vi "canDataSort.vi"() -> ()   [LabVIEW 2023] (continued)
8        68\t00\t97\tCC\t00\t19\t39\tFB\r\n      4502  1FFFFFFF   00000004    8        00\t00\tFF\tFF\tFF\tFF\tFF\tFF\r\n      4493  18F106A7   00000004    8        00\tF7\tFF\tFF\tFF\tFF\tFF\tCA\r\n      4492  1FFFFFFF   00000004    8        00\t20\tFF\tFF\tFF\tFF\tFF\tFF\r\n      4483  0CF102A7   00000004    8        30\t75\tE0\t2E\t80\tFF\tFF\tFD\r\n      4482  0CF101A7   00000004    8        68\t00\t97\tCC\t00\t19\t39\tFA\r\n      4482  1FFFFFFF   00000004    8        00\t00\tFF\tFF\tFF\tFF\tFF\tFF\r\n      4472  1FFFFFFF   00000004    8        00\t00\tFF\tFF\tFF\tFF\tFF\tFF\r\n      4463  0CF102A7   00000004    8        30\t75\tE0\t2E\t80\tFF\tFF\tFD\r\n      4463  0CF101A7   00000004    8        68\t00\t97\tCC\t00\t19\t39\tF9\r\n      4462  1FFFFFFF   00000004    8        00\t00\tFF\tFF\tFF\tFF\tFF\tFF\r\n      4503  0CF102A7   00000004    8        30\t75\tE0\t2E\t80\tFF\tFF\tFD\r\n      4503  0CF101A7   00000004    8        68\t00\t97\tCC\t00\t19\t39\tFB\r\n      4502  1FFFFFFF   00000004    8        00\t00\tFF\tFF\tFF\tFF\tFF\tFF\r\n      4493  18F106A7   00000004    8        00\tF7\tFF\tFF\tFF\tFF\tFF\tCA\r\n      4492  1FFFFFFF   00000004    8        00\t20\tFF\tFF\tFF\tFF\tFF\tFF\r\n      4483  0CF102A7   00000004    8        30\t75\tE0\t2E\t80\tFF\tFF\tFD\r\n      4482  0CF101A7   00000004    8        68\t00\t97\tCC\t00\t19\t39\tFA\r\n      4482  1FFFFFFF   00000004    8        00\t00\tFF\tFF\tFF\tFF\tFF\tFF\r\n      4472  1FFFFFFF   00000004    8        00\t00\tFF\tFF\tFF\tFF\tFF\tFF\r\n      4463  0CF102A7   00000004    8        30\t75\tE0\t2E\t80\tFF\tFF\tFD\r\n      4463  0CF101A7   00000004    8        68\t00\t97\tCC\t00\t19\t39\tF9\r\n      4512  1FFFFFFF   00000004    8        00\t00\tFF\tFF\tFF\tFF\tFF\tFF\r\n      4503  0CF102A7   00000004    8        30\t75\tE0\t2E\t80\tFF\tFF\tFD\r\n      4503  0CF101A7   00000004    8        68\t00\t97\tCC\t00\t19\t39\tFB\r\n      4502  1FFFFFFF   00000004    8        00\t00\tFF\tFF\tFF\tFF\tFF\tFF\r\n      4493  18F106A7   00000004    8        00\tF7\tFF\tFF\tFF\tFF\tFF\tCA\r\n      4492  1FFFFFFF   00000004    8        00\t20\tFF\tFF\tFF\tFF\tFF\tFF\r\n      4483  0CF102A7   00000004    8        30\t75\tE0\t2E\t80\tFF\tFF\tFD\r\n      4482  0CF101A7   00000004    8        68\t00\t97\tCC\t00\t19\t39\tFA\r\n      4482  1FFFFFFF   00000004    8        00\t00\tFF\tFF\tFF\tFF\tFF\tFF\r\n      4472  1FFFFFFF   00000004    8        00\t00\tFF\tFF\tFF\tFF\tFF\tFF\r\n      4463  0CF102A7   00000004    8        30\t75\tE0\t2E\t80\tFF\tFF\tFD\r\n      4522  1FFFFFFF   00000004    8        00\t00\tFF\tFF\tFF\tFF\tFF\tFF\r\n      4512  1FFFFFFF   00000004    8        00\t00\tFF\tFF\tFF\tFF\tFF\tFF\r\n      4503  0CF102A7   00000004    8        30\t75\tE0\t2E\t80\tFF\tFF\tFD\r\n      4503  0CF101A7   00000004    8        68\t00\t97\tCC\t00\t19\t39\tFB\r\n      4502  1FFFFFFF   00000004    8        00\t00\tFF\tFF\tFF\tFF\tFF\tFF\r\n      4493  18F106A7   00000004    8        00\tF7\tFF\tFF\tFF\tFF\tFF\tCA\r\n      4492  1FFFFFFF   00000004    8        00\t20\tFF\tFF\tFF\tFF\tFF\tFF\r\n      4483  0CF102A7   00000004    8        30\t75\tE0\t2E\t80\tFF\tFF\tFD\r\n      4482  0CF101A7   00000004    8        68\t00\t97\tCC\t00\t19\t39\tFA\r\n      4482  1FFFFFFF   00000004    8        00\t00\tFF\tFF\tFF\tFF\tFF\tFF\r\n      4472  1FFFFFFF   00000004    8        00\t00\tFF\tFF\tFF\tFF\tFF\tFF\r\n      4523  0CF101A7   00000004    8        68\t00\t97\tCC\t00\t19\t39\tFC\r\n      4522  1FFFFFFF   00000004    8        00\t00\tFF\tFF\tFF\tFF\tFF\tFF\r\n      4512  1FFFFFFF   00000004    8        00\t00\tFF\tFF\tFF\tFF\tFF\tFF\r\n      4503  0CF102A7   00000004    8        30\t75\tE0\t2E\t80\tFF\tFF\tFD\r\n      4503  0CF101A7   00000004    8        68\t00\t97\tCC\t00\t19\t39\tFB\r\n      4502  1FFFFFFF   00000004    8        00\t00\tFF\tFF\tFF\tFF\tFF\tFF\r\n      4493  18F106A7   00000004    8        00\tF7\tFF\tFF\tFF\tFF\tFF\tCA\r\n      4492  1FFFFFFF   00000004    8        00\t20\tFF\tFF\tFF\tFF\tFF\tFF\r\n      4483  0CF102A7   00000004    8        30\t75\tE0\t2E\t80\tFF\tFF\tFD\r\n      4482  0CF101A7   00000004    8        68\t00\t97\tCC\t00\t19\t39\tFA\r\n      4482  1FFFFFFF   00000004    8        00\t00\tFF\tFF\tFF\tFF\tFF\tFF\r\n      4523  0CF102A7   00000004    8        30\t75\tE0\t2E\t80\tFF\tFF\tFD\r\n      4523  0CF101A7   00000004    8        68\t00\t97\tCC\t00\t19\t39\tFC\r\n      4522  1FFFFFFF   00000004    8        00\t00\tFF\tFF\tFF\tFF\tFF\tFF\r\n      4512  1FFFFFFF   00000004    8        00\t00\tFF\tFF\tFF\tFF\tFF\tFF\r\n      4503  0CF102A7   00000004    8        30\t75\tE0\t2E\t80\tFF\tFF\tFD\r\n      4503  0CF101A7   00000004    8        68\t00\t97\tCC\t00\t19\t39\tFB\r\n      4502  1FFFFFFF   00000004    8        00\t00\tFF\tFF\tFF\tFF\tFF\tFF\r\n      4493  18F106A7   00000004    8        00\tF7\tFF\tFF\tFF\tFF\tFF\tCA\r\n      4492  1FFFFFFF   00000004    8        00\t20\tFF\tFF\tFF\tFF\tFF\tFF\r\n      4483  0CF102A7   00000004    8        30\t75\tE0\t2E\t80\tFF\tFF\tFD\r\n      4482  0CF101A7   00000004    8        68\t00\t97\tCC\t00\t19\t39\tFA\r\n      4532  1FFFFFFF   00000004    8        00\t20\tFF\tFF\tFF\tFF\tFF\tFF\r\n      4523  0CF102A7   00000004    8        30\t75\tE0\t2E\t80\tFF\tFF\tFD\r\n      4523  0CF101A7   00000004    8        68\t00\t97\tCC\t00\t19\t39\tFC\r\n      4522  1FFFFFFF   00000004    8        00\t00\tFF\tFF\tFF\tFF\tFF\tFF\r\n      4512  1FFFFFFF   00000004    8        00\t00\tFF\tFF\tFF\tFF\tFF\tFF\r\n      4503  0CF102A7   00000004    8        30\t75\tE0\t2E\t80\tFF\tFF\tFD\r\n      4503  0CF101A7   00000004    8        68\t00\t97\tCC\t00\t19\t39\tFB\r\n      4502  1FFFFFFF   00000004    8        00\t00\tFF\tFF\tFF\tFF\tFF\tFF\r\n      4493  18F106A7   00000004    8        00\tF7\tFF\tFF\tFF\tFF\tFF\tCA\r\n      4492  1FFFFFFF   00000004    8        00\t20\tFF\tFF\tFF\tFF\tFF\tFF\r\n      4483  0CF102A7   00000004    8        30\t75\tE0\t2E\t80\tFF\tFF\tFD\r\n      4541  18F11FF0   00000004    8        FF\t3F\t90\t68\t88\t1B\t10\t5C\r\n      4532  1FFFFFFF   00000004    8        00\t20\tFF\tFF\tFF\tFF\tFF\tFF\r\n      4523  0CF102A7   00000004    8        30\t75\tE0\t2E\t80\tFF\tFF\tFD\r\n      4523  0CF101A7   00000004    8        68\t00\t97\tCC\t00\t19\t39\tFC\r\n      4522  1FFFFFFF   00000004    8        00\t00\tFF\tFF\tFF\tFF\tFF\tFF\r\n      4512  1FFFFFFF   00000004    8        00\t00\tFF\tFF\tFF\tFF\tFF\tFF\r\n      4503  0CF102A7   00000004    8        30\t75\tE0\t2E\t80\tFF\tFF\tFD\r\n      4503  0CF101A7   00000004    8        68\t00\t97\tCC\t00\t19\t39\tFB\r\n      4502  1FFFFFFF   00000004    8        00\t00\tFF\tFF\tFF\tFF\tFF\tFF\r\n      4493  18F106A7   00000004    8        00\tF7\tFF\tFF\tFF\tFF\tFF\tCA\r\n      4492  1FFFFFFF   00000004    8        00\t20\tFF\tFF\tFF\tFF\tFF\tFF\r\n      4542  18F120F0   00000004    8        2B\t75\t60\tB1\tB0\t01\tFF\tFF\r\n      4541  18F11FF0   00000004    8        FF\t3F\t90\t68\t88\t1B\t10\t5C\r\n      4532  1FFFFFFF   00000004    8        00\t20\tFF\tFF\tFF\tFF\tFF\tFF\r\n      4523  0CF102A7   00000004    8        30\t75\tE0\t2E\t80\tFF\tFF\tFD\r\n      4523  0CF101A7   00000004    8        68\t00\t97\tCC\t00\t19\t39\tFC\r\n      4522  1FFFFFFF   00000004    8        00\t00\tFF\tFF\tFF\tFF\tFF\tFF\r\n      4512  1FFFFFFF   00000004    8        00\t00\tFF\tFF\tFF\tFF\tFF\tFF\r\n      4503  0CF102A7   00000004    8        30\t75\tE0\t2E\t80\tFF\tFF\tFD\r\n      4503  0CF101A7   00000004    8        68\t00\t97\tCC\t00\t19\t39\tFB\r\n      4502  1FFFFFFF   00000004    8        00\t00\tFF\tFF\tFF\tFF\tFF\tFF\r\n      4493  18F106A7   00000004    8        00\tF7\tFF\tFF\tFF\tFF\tFF\tCA\r\n      4542  0CF101A7   00000004    8        68\t00\t97\tCC\t00\t19\t39\tFD\r\n      4542  18F120F0   00000004    8        2B\t75\t60\tB1\tB0\t01\tFF\tFF\r\n      4541  18F11FF0   00000004    8        FF\t3F\t90\t68\t88\t1B\t10\t5C\r\n      4532  1FFFFFFF   00000004    8        00\t20\tFF\tFF\tFF\tFF\tFF\tFF\r\n      4523  0CF102A7   00000004    8        30\t75\tE0\t2E\t80\tFF\tFF\tFD\r\n      4523  0CF101A7   00000004    8        68\t00\t97\tCC\t00\t19\t39\tFC\r\n      4522  1FFFFFFF   00000004    8        00\t00\tFF\tFF\tFF\tFF\tFF\tFF\r\n      4512  1FFFFFFF   00000004    8        00\t00\tFF\tFF\tFF\tFF\tFF\tFF\r\n      4503  0CF102A7   00000004    8        30\t75\tE0\t2E\t80\tFF\tFF\tFD\r\n      4503  0CF101A7   00000004    8        68\t00\t97\tCC\t00\t19\t39\tFB\r\n      4502  1FFFFFFF   00000004    8        00\t00\tFF\tFF\tFF\tFF\tFF\tFF\r\n      4543  0C3C4D4A   00000004    8        BE\tFF\tFF\t7F\t18\tFF\tFF\t65\r\n      4542  0CF101A7   00000004    8        68\t00\t97\tCC\t00\t19\t39\tFD\r\n      4542  18F120F0   00000004    8        2B\t75\t60\tB1\tB0\t01\tFF\tFF\r\n      4541  18F11FF0   00000004    8        FF\t3F\t90\t68\t88\t1B\t10\t5C\r\n      4532  1FFFFFFF   00000004    8        00\t20\tFF\tFF\tFF\tFF\tFF\tFF\r\n      4523  0CF102A7   00000004    8        30\t75\tE0\t2E\t80\tFF\tFF\tFD\r\n      4523  0CF101A7   00000004    8        68\t00\t97\tCC\t00\t19\t39\tFC\r\n      4522  1FFFFFFF   00000004    8        00\t00\tFF\tFF\tFF\tFF\tFF\tFF\r\n      4512  1FFFFFFF   00000004    8        00\t00\tFF\tFF\tFF\tFF\tFF\tFF\r\n      4503  0CF102A7   00000004    8        30\t75\tE0\t2E\t80\tFF\tFF\tFD\r\n      4503  0CF101A7   00000004    8        68\t00\t97\tCC\t00\t19\t39\tFB\r\n      4544  0CF102A7   00000004    8        30\t75\tE0\t2E\t80\tFF\tFF\tFD\r\n      4543  0C3C4D4A   00000004    8        BE\tFF\tFF\t7F\t18\tFF\tFF\t65\r\n      4542  0CF101A7   00000004    8        68\t00\t97\tCC\t00\t19\t39\tFD\r\n      4542  18F120F0   00000004    8        2B\t75\t60\tB1\tB0\t01\tFF\tFF\r\n      4541  18F11FF0   00000004    8        FF\t3F\t90\t68\t88\t1B\t10\t5C\r\n      4532  1FFFFFFF   00000004    8        00\t20\tFF\tFF\tFF\tFF\tFF\tFF\r\n      4523  0CF102A7   00000004    8        30\t75\tE0\t2E\t80\tFF\tFF\tFD\r\n      4523  0CF101A7   00000004    8        68\t00\t97\tCC\t00\t19\t39\tFC\r\n      4522  1FFFFFFF   00000004    8        00\t00\tFF\tFF\tFF\tFF\tFF\tFF\r\n      4512  1FFFFFFF   00000004    8        00\t00\tFF\tFF\tFF\tFF\tFF\tFF\r\n      4503  0CF102A7   00000004    8        30\t75\tE0\t2E\t80\tFF\tFF\tFD\r\n      4544  0CF103A7   00000004    8        17\t1F\t08\t60\tB1\t1F\t08\t65\r\n      4544  0CF102A7   00000004    8        30\t75\tE0\t2E\t80\tFF\tFF\tFD\r\n      4543  0C3C4D4A   00000004    8        BE\tFF\tFF\t7F\t18\tFF\tFF\t65\r\n      4542  0CF101A7   00000004    8        68\t00\t97\tCC\t00\t19\t39\tFD\r\n      4542  18F120F0   00000004    8        2B\t75\t60\tB1\tB0\t01\tFF\tFF\r\n      4541  18F11FF0   00000004    8        FF\t3F\t90\t68\t88\t1B\t10\t5C\r\n      4532  1FFFFFFF   00000004    8        00\t20\tFF\tFF\tFF\tFF\tFF\tFF\r\n      4523  0CF102A7   00000004    8        30\t75\tE0\t2E\t80\tFF\tFF\tFD\r\n      4523  0CF101A7   00000004    8        68\t00\t97\tCC\t00\t19\t39\tFC\r\n      4522  1FFFFFFF   00000004    8        00\t00\tFF\tFF\tFF\tFF\tFF\tFF\r\n      4512  1FFFFFFF   00000004    8        00\t00\tFF\tFF\tFF\tFF\tFF\tFF\r\n      4545  0CF104A7   00000004    8        F0\t60\t22\tFC\tFF\tFF\tFF\t65\r\n      4544  0CF103A7   00000004    8        17\t1F\t08\t60\tB1\t1F\t08\t65\r\n      4544  0CF102A7   00000004    8        30\t75\tE0\t2E\t80\tFF\tFF\tFD\r\n      4543  0C3C4D4A   00000004    8        BE\tFF\tFF\t7F\t18\tFF\tFF\t65\r\n      4542  0CF101A7   00000004    8        68\t00\t97\tCC\t00\t19\t39\tFD\r\n      4542  18F120F0   00000004    8        2B\t75\t60\tB1\tB0\t01\tFF\tFF\r\n      4541  18F11FF0   00000004    8        FF\t3F\t90\t68\t88\t1B\t10\t5C\r\n      4532  1FFFFFFF   00000004    8        00\t20\tFF\tFF\tFF\tFF\tFF\tFF\r\n      4523  0CF102A7   00000004    8        30\t75\tE0\t2E\t80\tFF\tFF\tFD\r\n      4523  0CF101A7   00000004    8        68\t00\t97\tCC\t00\t19\t39\tFC\r\n      4522  1FFFFFFF   00000004    8        00\t00\tFF\tFF\tFF\tFF\tFF\tFF\r\n      4545  18F106A7   00000004    8        00\tF7\tFF\tFF\tFF\tFF\tFF\tCB\r\n      4545  0CF104A7   00000004    8        F0\t60\t22\tFC\tFF\tFF\tFF\t65\r\n      4544  0CF103A7   00000004    8        17\t1F\t08\t60\tB1\t1F\t08\t65\r\n      4544  0CF102A7   00000004    8        30\t75\tE0\t2E\t80\tFF\tFF\tFD\r\n      4543  0C3C4D4A   00000004    8        BE\tFF\tFF\t7F\t18\tFF\tFF\t65\r\n      4542  0CF101A7   00000004    8        68\t00\t97\tCC\t00\t19\t39\tFD\r\n      4542  18F120F0   00000004    8        2B\t75\t60\tB1\tB0\t01\tFF\tFF\r\n      4541  18F11FF0   00000004    8        FF\t3F\t90\t68\t88\t1B\t10\t5C\r\n      4532  1FFFFFFF   00000004    8        00\t20\tFF\tFF\tFF\tFF\tFF\tFF\r\n      4523  0CF102A7   00000004    8        30\t75\tE0\t2E\t80\tFF\tFF\tFD\r\n      4523  0CF101A7   00000004    8        68\t00\t97\tCC\t00\t19\t39\tFC\r\n      4546  18F121F0   00000004    8        09\t34\t00\t00\tFF\tFF\tB0\t01\r\n      4545  18F106A7   00000004    8        00\tF7\tFF\tFF\tFF\tFF\tFF\tCB\r\n      4545  0CF104A7   00000004    8        F0\t60\t22\tFC\tFF\tFF\tFF\t65\r\n      4544  0CF103A7   00000004    8        17\t1F\t08\t60\tB1\t1F\t08\t65\r\n      4544  0CF102A7   00000004    8        30\t75\tE0\t2E\t80\tFF\tFF\tFD\r\n      4543  0C3C4D4A   00000004    8        BE\tFF\tFF\t7F\t18\tFF\tFF\t65\r\n      4542  0CF101A7   00000004    8        68\t00\t97\tCC\t00\t19\t39\tFD\r\n      4542  18F120F0   00000004    8        2B\t75\t60\tB1\tB0\t01\tFF\tFF\r\n      4541  18F11FF0   00000004    8        FF\t3F\t90\t68\t88\t1B\t10\t5C\r\n      4532  1FFFFFFF   00000004    8        00\t20\tFF\tFF\tFF\tFF\tFF\tFF\r\n      4523  0CF102A7   00000004    8        30\t75\tE0\t2E\t80\tFF\tFF\tFD\r\n      4546  1FFFFFFF   00000004    8        00\t00\tFF\tFF\tFF\tFF\tFF\tFF\r\n      4546  18F121F0   00000004    8        09\t34\t00\t00\tFF\tFF\tB0\t01\r\n      4545  18F106A7   00000004    8        00\tF7\tFF\tFF\tFF\tFF\tFF\tCB\r\n      4545  0CF104A7   00000004    8        F0\t60\t22\tFC\tFF\tFF\tFF\t65\r\n      4544  0CF103A7   00000004    8        17\t1F\t08\t60\tB1\t1F\t08\t65\r\n      4544  0CF102A7   00000004    8        30\t75\tE0\t2E\t80\tFF\tFF\tFD\r\n      4543  0C3C4D4A   00000004    8        BE\tFF\tFF\t7F\t18\tFF\tFF\t65\r\n      4542  0CF101A7   00000004    8        68\t00\t97\tCC\t00\t19\t39\tFD\r\n      4542  18F120F0   00000004    8        2B\t75\t60\tB1\tB0\t01\tFF\tFF\r\n      4541  18F11FF0   00000004    8        FF\t3F\t90\t68\t88\t1B\t10\t5C\r\n      4532  1FFFFFFF   00000004    8        00\t20\tFF\tFF\tFF\tFF\tFF\tFF\r\n      4552  1FFFFFFF   00000004    8        00\t00\tFF\tFF\tFF\tFF\tFF\tFF\r\n      4546  1FFFFFFF   00000004    8        00\t00\tFF\tFF\tFF\tFF\tFF\tFF\r\n      4546  18F121F0   00000004    8        09\t34\t00\t00\tFF\tFF\tB0\t01\r\n      4545  18F106A7   00000004    8        00\tF7\tFF\tFF\tFF\tFF\tFF\tCB\r\n      4545  0CF104A7   00000004    8        F0\t60\t22\tFC\tFF\tFF\tFF\t65\r\n      4544  0CF103A7   00000004    8        17\t1F\t08\t60\tB1\t1F\t08\t65\r\n      4544  0CF102A7   00000004    8        30\t75\tE0\t2E\t80\tFF\tFF\tFD\r\n      4543  0C3C4D4A   00000004    8        BE\tFF\tFF\t7F\t18\tFF\tFF\t65\r\n      4542  0CF101A7   00000004    8        68\t00\t97\tCC\t00\t19\t39\tFD\r\n      4542  18F120F0   00000004    8        2B\t75\t60\tB1\tB0\t01\tFF\tFF\r\n      4541  18F11FF0   00000004    8        FF\t3F\t90\t68\t88\t1B\t10\t5C\r\n      4562  1FFFFFFF   00000004    8        00\t00\tFF\tFF\tFF\tFF\tFF\tFF\r\n      4552  1FFFFFFF   00000004    8        00\t00\tFF\tFF\tFF\tFF\tFF\tFF\r\n      4546  1FFFFFFF   00000004    8        00\t00\tFF\tFF\tFF\tFF\tFF\tFF\r\n      4546  18F121F0   00000004    8        09\t34\t00\t00\tFF\tFF\tB0\t01\r\n      4545  18F106A7   00000004    8        00\tF7\tFF\tFF\tFF\tFF\tFF\tCB\r\n      4545  0CF104A7   00000004    8        F0\t60\t22\tFC\tFF\tFF\tFF\t65\r\n      4544  0CF103A7   00000004    8        17\t1F\t08\t60\tB1\t1F\t08\t65\r\n      4544  0CF102A7   00000004    8        30\t75\tE0\t2E\t80\tFF\tFF\tFD\r\n      4543  0C3C4D4A   00000004    8        BE\tFF\tFF\t7F\t18\tFF\tFF\t65\r\n      4542  0CF101A7   00000004    8        68\t00\t97\tCC\t00\t19\t39\tFD\r\n      4542  18F120F0   00000004    8        2B\t75\t60\tB1\tB0\t01\tFF\tFF\r\n      4563  0CF101A7   00000004    8        68\t00\t97\tCC\t00\t19\t39\tFE\r\n      4562  1FFFFFFF   00000004    8        00\t00\tFF\tFF\tFF\tFF\tFF\tFF\r\n      4552  1FFFFFFF   00000004    8        00\t00\tFF\tFF\tFF\tFF\tFF\tFF\r\n      4546  1FFFFFFF   00000004    8        00\t00\tFF\tFF\tFF\tFF\tFF\tFF\r\n      4546  18F121F0   00000004    8        09\t34\t00\t00\tFF\tFF\tB0\t01\r\n      4545  18F106A7   00000004    8        00\tF7\tFF\tFF\tFF\tFF\tFF\tCB\r\n      4545  0CF104A7   00000004    8        F0\t60\t22\tFC\tFF\tFF\tFF\t65\r\n      4544  0CF103A7   00000004    8        17\t1F\t08\t60\tB1\t1F\t08\t65\r\n      4544  0CF102A7   00000004    8        30\t75\tE0\t2E\t80\tFF\tFF\tFD\r\n      4543  0C3C4D4A   00000004    8        BE\tFF\tFF\t7F\t18\tFF\tFF\t65\r\n      4542  0CF101A7   00000004    8        68\t00\t97\tCC\t00\t19\t39\tFD\r\n      4563  0CF102A7   00000004    8        30\t75\tE0\t2E\t80\tFF\tFF\tFD\r\n      4563  0CF101A7   00000004    8        68\t00\t97\tCC\t00\t19\t39\tFE\r\n      4562  1FFFFFFF   00000004    8        00\t00\tFF\tFF\tFF\tFF\tFF\tFF\r\n      4552  1FFFFFFF   00000004    8        00\t00\tFF\tFF\tFF\tFF\tFF\tFF\r\n      4546  1FFFFFFF   00000004    8        00\t00\tFF\tFF\tFF\tFF\tFF\tFF\r\n      4546  18F121F0   00000004    8        09\t34\t00\t00\tFF\tFF\tB0\t01\r\n      4545  18F106A7   00000004    8        00\tF7\tFF\tFF\tFF\tFF\tFF\tCB\r\n      4545  0CF104A7   00000004    8        F0\t60\t22\tFC\tFF\tFF\tFF\t65\r\n      4544  0CF103A7   00000004    8        17\t1F\t08\t60\tB1\t1F\t08\t65\r\n      4544  0CF102A7   00000004    8        30\t75\tE0\t2E\t80\tFF\tFF\tFD\r\n      4543  0C3C4D4A   00000004    8        BE\tFF\tFF\t7F\t18\tFF\tFF\t65\r\n      4572  1FFFFFFF   00000004    8        00\t00\tFF\tFF\tFF\tFF\tFF\tFF\r\n      4563  0CF102A7   00000004    8        30\t75\tE0\t2E\t80\tFF\tFF\tFD\r\n      4563  0CF101A7   00000004    8        68\t00\t97\tCC\t00\t19\t39\tFE\r\n      4562  1FFFFFFF   00000004    8        00\t00\tFF\tFF\tFF\tFF\tFF\tFF\r\n      4552  1FFFFFFF   00000004    8        00\t00\tFF\tFF\tFF\tFF\tFF\tFF\r\n      4546  1FFFFFFF   00000004    8        00\t00\tFF\tFF\tFF\tFF\tFF\tFF\r\n      4546  18F121F0   00000004    8        09\t34\t00\t00\tFF\tFF\tB0\t01\r\n      4545  18F106A7   00000004    8        00\tF7\tFF\tFF\tFF\tFF\tFF\tCB\r\n      4545  0CF104A7   00000004    8        F0\t60\t22\tFC\tFF\tFF\tFF\t65\r\n      4544  0CF103A7   00000004    8        17\t1F\t08\t60\tB1\t1F\t08\t65\r\n      4544  0CF102A7   00000004    8        30\t75\tE0\t2E\t80\tFF\tFF\tFD\r\n      4582  1FFFFFFF   00000004    8        00\t00\tFF\tFF\tFF\tFF\tFF\tFF\r\n      4572  1FFFFFFF   00000004    8        00\t00\tFF\tFF\tFF\tFF\tFF\tFF\r\n      4563  0CF102A7   00000004    8        30\t75\tE0\t2E\t80\tFF\tFF\tFD\r\n      4563  0CF101A7   00000004    8        68\t00\t97\tCC\t00\t19\t39\tFE\r\n      4562  1FFFFFFF   00000004    8        00\t00\tFF\tFF\tFF\tFF\tFF\tFF\r\n      4552  1FFFFFFF   00000004    8        00\t00\tFF\tFF\tFF\tFF\tFF\tFF\r\n      4546  1FFFFFFF   00000004    8        00\t00\tFF\tFF\tFF\tFF\tFF\tFF\r\n      4546  18F121F0   00000004    8        09\t34\t00\t00\tFF\tFF\tB0\t01\r\n      4545  18F106A7   00000004    8        00\tF7\tFF\tFF\tFF\tFF\tFF\tCB\r\n      4545  0CF104A7   00000004    8        F0\t60\t22\tFC\tFF\tFF\tFF\t65\r\n      4544  0CF103A7   00000004    8        17\t1F\t08\t60\tB1\t1F\t08\t65\r\n      4583  0CF101A7   00000004    8        68\t00\t97\tCC\t00\t19\t39\tFF\r\n      4582  1FFFFFFF   00000004    8        00\t00\tFF\tFF\tFF\tFF\tFF\tFF\r\n      4572  1FFFFFFF   00000004    8        00\t00\tFF\tFF\tFF\tFF\tFF\tFF\r\n      4563  0CF102A7   00000004    8        30\t75\tE0\t2E\t80\tFF\tFF\tFD\r\n      4563  0CF101A7   00000004    8        68\t00\t97\tCC\t00\t19\t39\tFE\r\n      4562  1FFFFFFF   00000004    8        00\t00\tFF\tFF\tFF\tFF\tFF\tFF\r\n      4552  1FFFFFFF   00000004    8        00\t00\tFF\tFF\tFF\tFF\tFF\tFF\r\n      4546  1FFFFFFF   00000004    8        00\t00\tFF\tFF\tFF\tFF\tFF\tFF\r\n      4546  18F121F0   00000004    8        09\t34\t00\t00\tFF\tFF\tB0\t01\r\n      4545  18F106A7   00000004    8        00\tF7\tFF\tFF\tFF\tFF\tFF\tCB\r\n      4545  0CF104A7   00000004    8        F0\t60\t22\tFC\tFF\tFF\tFF\t65\r\n      4583  0CF102A7   00000004    8        30\t75\tE0\t2E\t80\tFF\tFF\tFD\r\n      4583  0CF101A7   00000004    8        68\t00\t97\tCC\t00\t19\t39\tFF\r\n      4582  1FFFFFFF   00000004    8        00\t00\tFF\tFF\tFF\tFF\tFF\tFF\r\n      4572  1FFFFFFF   00000004    8        00\t00\tFF\tFF\tFF\tFF\tFF\tFF\r\n      4563  0CF102A7   00000004    8        30\t75\tE0\t2E\t80\tFF\tFF\tFD\r\n      4563  0CF101A7   00000004    8        68\t00\t97\tCC\t00\t19\t39\tFE\r\n      4562  1FFFFFFF   00000004    8        00\t00\tFF\tFF\tFF\tFF\tFF\tFF\r\n      4552  1FFFFFFF   00000004    8        00\t00\tFF\tFF\tFF\tFF\tFF\tFF\r\n      4546  1FFFFFFF   00000004    8        00\t00\tFF\tFF\tFF\tFF\tFF\tFF\r\n      4546  18F121F0   00000004    8        09\t34\t00\t00\tFF\tFF\tB0\t01\r\n      4545  18F106A7   00000004    8        00\tF7\tFF\tFF\tFF\tFF\tFF\tCB\r\n      4592  1FFFFFFF   00000004    8        00\t00\tFF\tFF\tFF\tFF\tFF\tFF\r\n      4583  0CF102A7   00000004    8        30\t75\tE0\t2E\t80\tFF\tFF\tFD\r\n      4583  0CF101A7   00000004    8        68\t00\t97\tCC\t00\t19\t39\tFF\r\n      4582  1FFFFFFF   00000004    8        00\t00\tFF\tFF\tFF\tFF\tFF\tFF\r\n      4572  1FFFFFFF   00000004    8        00\t00\tFF\tFF\tFF\tFF\tFF\tFF\r\n      4563  0CF102A7   00000004    8        30\t75\tE0\t2E\t80\tFF\tFF\tFD\r\n      4563  0CF101A7   00000004    8        68\t00\t97\tCC\t00\t19\t39\tFE\r\n      4562  1FFFFFFF   00000004    8        00\t00\tFF\tFF\tFF\tFF\tFF\tFF\r\n      4552  1FFFFFFF   00000004    8        00\t00\tFF\tFF\tFF\tFF\tFF\tFF\r\n      4546  1FFFFFFF   00000004    8        00\t00\tFF\tFF\tFF\tFF\tFF\tFF\r\n      4546  18F121F0   00000004    8        09\t34\t00\t00\tFF\tFF\tB0\t01\r\n      4593  18F106A7   00000004    8        00\tF7\tFF\tFF\tFF\tFF\tFF\tCC\r\n      4592  1FFFFFFF   00000004    8        00\t00\tFF\tFF\tFF\tFF\tFF\tFF\r\n      4583  0CF102A7   00000004    8        30\t75\tE0\t2E\t80\tFF\tFF\tFD\r\n      4583  0CF101A7   00000004    8        68\t00\t97\tCC\t00\t19\t39\tFF\r\n      4582  1FFFFFFF   00000004    8        00\t00\tFF\tFF\tFF\tFF\tFF\tFF\r\n      4572  1FFFFFFF   00000004    8        00\t00\tFF\tFF\tFF\tFF\tFF\tFF\r\n      4563  0CF102A7   00000004    8        30\t75\tE0\t2E\t80\tFF\tFF\tFD\r\n      4563  0CF101A7   00000004    8        68\t00\t97\tCC\t00\t19\t39\tFE\r\n      4562  1FFFFFFF   00000004    8        00\t00\tFF\tFF\tFF\tFF\tFF\tFF\r\n      4552  1FFFFFFF   00000004    8        00\t00\tFF\tFF\tFF\tFF\tFF\tFF\r\n      4546  1FFFFFFF   00000004    8        00\t00\tFF\tFF\tFF\tFF\tFF\tFF\r\n      4602  1FFFFFFF   00000004    8        00\t00\tFF\tFF\tFF\tFF\tFF\tFF\r\n      4593  18F106A7   00000004    8        00\tF7\tFF\tFF\tFF\tFF\tFF\tCC\r\n      4592  1FFFFFFF   00000004    8        00\t00\tFF\tFF\tFF\tFF\tFF\tFF\r\n      4583  0CF102A7   00000004    8        30\t75\tE0\t2E\t80\tFF\tFF\tFD\r\n      4583  0CF101A7   00000004    8        68\t00\t97\tCC\t00\t19\t39\tFF\r\n      4582  1FFFFFFF   00000004    8        00\t00\tFF\tFF\tFF\tFF\tFF\tFF\r\n      4572  1FFFFFFF   00000004    8        00\t00\tFF\tFF\tFF\tFF\tFF\tFF\r\n      4563  0CF102A7   00000004    8        30\t75\tE0\t2E\t80\tFF\tFF\tFD\r\n      4563  0CF101A7   00000004    8        68\t00\t97\tCC\t00\t19\t39\tFE\r\n      4562  1FFFFFFF   00000004    8        00\t00\tFF\tFF\tFF\tFF\tFF\tFF\r\n      4552  1FFFFFFF   00000004    8        00\t00\tFF\tFF\tFF\tFF\tFF\tFF\r\n      4603  0CF101A7   00000004    8        68\t00\t97\tCC\t00\t19\t39\t00\r\n      4602  1FFFFFFF   00000004    8        00\t00\tFF\tFF\tFF\tFF\tFF\tFF\r\n      4593  18F106A7   00000004    8        00\tF7\tFF\tFF\tFF\tFF\tFF\tCC\r\n      4592  1FFFFFFF   00000004    8        00\t00\tFF\tFF\tFF\tFF\tFF\tFF\r\n      4583  0CF102A7   00000004    8        30\t75\tE0\t2E\t80\tFF\tFF\tFD\r\n      4583  0CF101A7   00000004    8        68\t00\t97\tCC\t00\t19\t39\tFF\r\n      4582  1FFFFFFF   00000004    8        00\t00\tFF\tFF\tFF\tFF\tFF\tFF\r\n      4572  1FFFFFFF   00000004    8        00\t00\tFF\tFF\tFF\tFF\tFF\tFF\r\n      4563  0CF102A7   00000004    8        30\t75\tE0\t2E\t80\tFF\tFF\tFD\r\n      4563  0CF101A7   00000004    8        68\t00\t97\tCC\t00\t19\t39\tFE\r\n      4562  1FFFFFFF   00000004    8        00\t00\tFF\tFF\tFF\tFF\tFF\tFF\r\n      4603  0CF102A7   00000004    8        30\t75\tE0\t2E\t80\tFF\tFF\tFD\r\n      4603  0CF101A7   00000004    8        68\t00\t97\tCC\t00\t19\t39\t00\r\n      4602  1FFFFFFF   00000004    8        00\t00\tFF\tFF\tFF\tFF\tFF\tFF\r\n      4593  18F106A7   00000004    8        00\tF7\tFF\tFF\tFF\tFF\tFF\tCC\r\n      4592  1FFFFFFF   00000004    8        00\t00\tFF\tFF\tFF\tFF\tFF\tFF\r\n      4583  0CF102A7   00000004    8        30\t75\tE0\t2E\t80\tFF\tFF\tFD\r\n      4583  0CF101A7   00000004    8        68\t00\t97\tCC\t00\t19\t39\tFF\r\n      4582  1FFFFFFF   00000004    8        00\t00\tFF\tFF\tFF\tFF\tFF\tFF\r\n      4572  1FFFFFFF   00000004    8        00\t00\tFF\tFF\tFF\tFF\tFF\tFF\r\n      4563  0CF102A7   00000004    8        30\t75\tE0\t2E\t80\tFF\tFF\tFD\r\n      4563  0CF101A7   00000004    8        68\t00\t97\tCC\t00\t19\t39\tFE\r\n      4612  1FFFFFFF   00000004    8        00\t00\tFF\tFF\tFF\tFF\tFF\tFF\r\n      4603  0CF102A7   00000004    8        30\t75\tE0\t2E\t80\tFF\tFF\tFD\r\n      4603  0CF101A7   00000004    8        68\t00\t97\tCC\t00\t19\t39\t00\r\n      4602  1FFFFFFF   00000004    8        00\t00\tFF\tFF\tFF\tFF\tFF\tFF\r\n      4593  18F106A7   00000004    8        00\tF7\tFF\tFF\tFF\tFF\tFF\tCC\r\n      4592  1FFFFFFF   00000004    8        00\t00\tFF\tFF\tFF\tFF\tFF\tFF\r\n      4583  0CF102A7   00000004    8        30\t75\tE0\t2E\t80\tFF\tFF\tFD\r\n      4583  0CF101A7   00000004    8        68\t00\t97\tCC\t00\t19\t39\tFF\r\n      4582  1FFFFFFF   00000004    8        00\t00\tFF\tFF\tFF\tFF\tFF\tFF\r\n      4572  1FFFFFFF   00000004    8        00\t00\tFF\tFF\tFF\tFF\tFF\tFF\r\n      4563  0CF102A7   00000004    8        30\t75\tE0\t2E\t80\tFF\tFF\tFD\r\n      4622  1FFFFFFF   00000004    8        00\t00\tFF\tFF\tFF\tFF\tFF\tFF\r\n      4612  1FFFFFFF   00000004    8        00\t00\tFF\tFF\tFF\tFF\tFF\tFF\r\n      4603  0CF102A7   00000004    8        30\t75\tE0\t2E\t80\tFF\tFF\tFD\r\n      4603  0CF101A7   00000004    8        68\t00\t97\tCC\t00\t19\t39\t00\r\n      4602  1FFFFFFF   00000004    8        00\t00\tFF\tFF\tFF\tFF\tFF\tFF\r\n      4593  18F106A7   00000004    8        00\tF7\tFF\tFF\tFF\tFF\tFF\tCC\r\n      4592  1FFFFFFF   00000004    8        00\t00\tFF\tFF\tFF\tFF\tFF\tFF\r\n      4583  0CF102A7   00000004    8        30\t75\tE0\t2E\t80\tFF\tFF\tFD\r\n      4583  0CF101A7   00000004    8        68\t00\t97\tCC\t00\t19\t39\tFF\r\n      4582  1FFFFFFF   00000004    8        00\t00\tFF\tFF\tFF\tFF\tFF\tFF\r\n      4572  1FFFFFFF   00000004    8        00\t00\tFF\tFF\tFF\tFF\tFF\tFF\r\n      4623  0CF101A7   00000004    8        68\t00\t97\tCC\t00\t19\t39\t01\r\n      4622  1FFFFFFF   00000004    8        00\t00\tFF\tFF\tFF\tFF\tFF\tFF\r\n      4612  1FFFFFFF   00000004    8        00\t00\tFF\tFF\tFF\tFF\tFF\tFF\r\n      4603  0CF102A7   00000004    8        30\t75\tE0\t2E\t80\tFF\tFF\tFD\r\n      4603  0CF101A7   00000004    8        68\t00\t97\tCC\t00\t19\t39\t00\r\n      4602  1FFFFFFF   00000004    8        00\t00\tFF\tFF\tFF\tFF\tFF\tFF\r\n      4593  18F106A7   00000004    8        00\tF7\tFF\tFF\tFF\tFF\tFF\tCC\r\n      4592  1FFFFFFF   00000004    8        00\t00\tFF\tFF\tFF\tFF\tFF\tFF\r\n      4583  0CF102A7   00000004    8        30\t75\tE0\t2E\t80\tFF\tFF\tFD\r\n      4583  0CF101A7   00000004    8        68\t00\t97\tCC\t00\t19\t39\tFF\r\n      4582  1FFFFFFF   00000004    8        00\t00\tFF\tFF\tFF\tFF\tFF\tFF\r\n      4623  0CF102A7   00000004    8        30\t75\tE0\t2E\t80\tFF\tFF\tFD\r\n      4623  0CF101A7   00000004    8        68\t00\t97\tCC\t00\t19\t39\t01\r\n      4622  1FFFFFFF   00000004    8        00\t00\tFF\tFF\tFF\tFF\tFF\tFF\r\n      4612  1FFFFFFF   00000004    8        00\t00\tFF\tFF\tFF\tFF\tFF\tFF\r\n      4603  0CF102A7   00000004    8        30\t75\tE0\t2E\t80\tFF\tFF\tFD\r\n      4603  0CF101A7   00000004    8        68\t00\t97\tCC\t00\t19\t39\t00\r\n      4602  1FFFFFFF   00000004    8        00\t00\tFF\tFF\tFF\tFF\tFF\tFF\r\n      4593  18F106A7   00000004    8        00\tF7\tFF\tFF\tFF\tFF\tFF\tCC\r\n      4592  1FFFFFFF   00000004    8        00\t00\tFF\tFF\tFF\tFF\tFF\tFF\r\n      4583  0CF102A7   00000004    8        30\t75\tE0\t2E\t80\tFF\tFF\tFD\r\n      4583  0CF101A7   00000004    8        68\t00\t97\tCC\t00\t19\t39\tFF\r\n      4632  1FFFFFFF   00000004    8        00\t00\tFF\tFF\tFF\tFF\tFF\tFF\r\n      4623  0CF102A7   00000004    8        30\t75\tE0\t2E\t80\tFF\tFF\tFD\r\n      4623  0CF101A7   00000004    8        68\t00\t97\tCC\t00\t19\t39\t01\r\n      4622  1FFFFFFF   00000004    8        00\t00\tFF\tFF\tFF\tFF\tFF\tFF\r\n      4612  1FFFFFFF   00000004    8        00\t00\tFF\tFF\tFF\tFF\tFF\tFF\r\n      4603  0CF102A7   00000004    8        30\t75\tE0\t2E\t80\tFF\tFF\tFD\r\n      4603  0CF101A7   00000004    8        68\t00\t97\tCC\t00\t19\t39\t00\r\n      4602  1FFFFFFF   00000004    8        00\t00\tFF\tFF\tFF\tFF\tFF\tFF\r\n      4593  18F106A7   00000004    8        00\tF7\tFF\tFF\tFF\tFF\tFF\tCC\r\n      4592  1FFFFFFF   00000004    8        00\t00\tFF\tFF\tFF\tFF\tFF\tFF\r\n      4583  0CF102A7   00000004    8        30\t75\tE0\t2E\t80\tFF\tFF\tFD\r\n      4642  18F11FF0   00000004    8        FF\t3F\t90\t68\t88\t1B\t10\t6C\r\n      4632  1FFFFFFF   00000004    8        00\t00\tFF\tFF\tFF\tFF\tFF\tFF\r\n      4623  0CF102A7   00000004    8        30\t75\tE0\t2E\t80\tFF\tFF\tFD\r\n      4623  0CF101A7   00000004    8        68\t00\t97\tCC\t00\t19\t39\t01\r\n      4622  1FFFFFFF   00000004    8        00\t00\tFF\tFF\tFF\tFF\tFF\tFF\r\n      4612  1FFFFFFF   00000004    8        00\t00\tFF\tFF\tFF\tFF\tFF\tFF\r\n      4603  0CF102A7   00000004    8        30\t75\tE0\t2E\t80\tFF\tFF\tFD\r\n      4603  0CF101A7   00000004    8        68\t00\t97\tCC\t00\t19\t39\t00\r\n      4602  1FFFFFFF   00000004    8        00\t00\tFF\tFF\tFF\tFF\tFF\tFF\r\n      4593  18F106A7   00000004    8        00\tF7\tFF\tFF\tFF\tFF\tFF\tCC\r\n      4592  1FFFFFFF   00000004    8        00\t00\tFF\tFF\tFF\tFF\tFF\tFF\r\n      4642  0CF101A7   00000004    8        68\t00\t97\tCC\t00\t19\t39\t02\r\n      4642  18F11FF0   00000004    8        FF\t3F\t90\t68\t88\t1B\t10\t6C\r\n      4632  1FFFFFFF   00000004    8        00\t00\tFF\tFF\tFF\tFF\tFF\tFF\r\n      4623  0CF102A7   00000004    8        30\t75\tE0\t2E\t80\tFF\tFF\tFD\r\n      4623  0CF101A7   00000004    8        68\t00\t97\tCC\t00\t19\t39\t01\r\n      4622  1FFFFFFF   00000004    8        00\t00\tFF\tFF\tFF\tFF\tFF\tFF\r\n      4612  1FFFFFFF   00000004    8        00\t00\tFF\tFF\tFF\tFF\tFF\tFF\r\n      4603  0CF102A7   00000004    8        30\t75\tE0\t2E\t80\tFF\tFF\tFD\r\n      4603  0CF101A7   00000004    8        68\t00\t97\tCC\t00\t19\t39\t00\r\n      4602  1FFFFFFF   00000004    8        00\t00\tFF\tFF\tFF\tFF\tFF\tFF\r\n      4593  18F106A7   00000004    8        00\tF7\tFF\tFF\tFF\tFF\tFF\tCC\r\n      4643  0CF102A7   00000004    8        30\t75\tE0\t2E\t80\tFF\tFF\tFD\r\n      4642  0CF101A7   00000004    8        68\t00\t97\tCC\t00\t19\t39\t02\r\n      4642  18F11FF0   00000004    8        FF\t3F\t90\t68\t88\t1B\t10\t6C\r\n      4632  1FFFFFFF   00000004    8        00\t00\tFF\tFF\tFF\tFF\tFF\tFF\r\n      4623  0CF102A7   00000004    8        30\t75\tE0\t2E\t80\tFF\tFF\tFD\r\n      4623  0CF101A7   00000004    8        68\t00\t97\tCC\t00\t19\t39\t01\r\n      4622  1FFFFFFF   00000004    8        00\t00\tFF\tFF\tFF\tFF\tFF\tFF\r\n      4612  1FFFFFFF   00000004    8        00\t00\tFF\tFF\tFF\tFF\tFF\tFF\r\n      4603  0CF102A7   00000004    8        30\t75\tE0\t2E\t80\tFF\tFF\tFD\r\n      4603  0CF101A7   00000004    8        68\t00\t97\tCC\t00\t19\t39\t00\r\n      4602  1FFFFFFF   00000004    8        00\t00\tFF\tFF\tFF\tFF\tFF\tFF\r\n      4644  0C3C4D4A   00000004    8        BE\tFF\tFF\t7F\t18\tFF\tFF\t66\r\n      4643  0CF102A7   00000004    8        30\t75\tE0\t2E\t80\tFF\tFF\tFD\r\n      4642  0CF101A7   00000004    8        68\t00\t97\tCC\t00\t19\t39\t02\r\n      4642  18F11FF0   00000004    8        FF\t3F\t90\t68\t88\t1B\t10\t6C\r\n      4632  1FFFFFFF   00000004    8        00\t00\tFF\tFF\tFF\tFF\tFF\tFF\r\n      4623  0CF102A7   00000004    8        30\t75\tE0\t2E\t80\tFF\tFF\tFD\r\n      4623  0CF101A7   00000004    8        68\t00\t97\tCC\t00\t19\t39\t01\r\n      4622  1FFFFFFF   00000004    8        00\t00\tFF\tFF\tFF\tFF\tFF\tFF\r\n      4612  1FFFFFFF   00000004    8        00\t00\tFF\tFF\tFF\tFF\tFF\tFF\r\n      4603  0CF102A7   00000004    8        30\t75\tE0\t2E\t80\tFF\tFF\tFD\r\n      4603  0CF101A7   00000004    8        68\t00\t97\tCC\t00\t19\t39\t00\r\n      4644  0CF103A7   00000004    8        17\t1F\t08\t60\tB1\t1F\t08\t66\r\n      4644  0C3C4D4A   00000004    8        BE\tFF\tFF\t7F\t18\tFF\tFF\t66\r\n      4643  0CF102A7   00000004    8        30\t75\tE0\t2E\t80\tFF\tFF\tFD\r\n      4642  0CF101A7   00000004    8        68\t00\t97\tCC\t00\t19\t39\t02\r\n      4642  18F11FF0   00000004    8        FF\t3F\t90\t68\t88\t1B\t10\t6C\r\n      4632  1FFFFFFF   00000004    8        00\t00\tFF\tFF\tFF\tFF\tFF\tFF\r\n      4623  0CF102A7   00000004    8        30\t75\tE0\t2E\t80\tFF\tFF\tFD\r\n      4623  0CF101A7   00000004    8        68\t00\t97\tCC\t00\t19\t39\t01\r\n      4622  1FFFFFFF   00000004    8        00\t00\tFF\tFF\tFF\tFF\tFF\tFF\r\n      4612  1FFFFFFF   00000004    8        00\t00\tFF\tFF\tFF\tFF\tFF\tFF\r\n      4603  0CF102A7   00000004    8        30\t75\tE0\t2E\t80\tFF\tFF\tFD\r\n      4645  0CF104A7   00000004    8        F0\t60\t22\tFC\tFF\tFF\tFF\t66\r\n      4644  0CF103A7   00000004    8        17\t1F\t08\t60\tB1\t1F\t08\t66\r\n      4644  0C3C4D4A   00000004    8        BE\tFF\tFF\t7F\t18\tFF\tFF\t66\r\n      4643  0CF102A7   00000004    8        30\t75\tE0\t2E\t80\tFF\tFF\tFD\r\n      4642  0CF101A7   00000004    8        68\t00\t97\tCC\t00\t19\t39\t02\r\n      4642  18F11FF0   00000004    8        FF\t3F\t90\t68\t88\t1B\t10\t6C\r\n      4632  1FFFFFFF   00000004    8        00\t00\tFF\tFF\tFF\tFF\tFF\tFF\r\n      4623  0CF102A7   00000004    8        30\t75\tE0\t2E\t80\tFF\tFF\tFD\r\n      4623  0CF101A7   00000004    8        68\t00\t97\tCC\t00\t19\t39\t01\r\n      4622  1FFFFFFF   00000004    8        00\t00\tFF\tFF\tFF\tFF\tFF\tFF\r\n      4612  1FFFFFFF   00000004    8        00\t00\tFF\tFF\tFF\tFF\tFF\tFF\r\n      4645  0CF105A7   00000004    8        94\t11\t00\t55\tFF\tFF\tFF\t23\r\n      4645  0CF104A7   00000004    8        F0\t60\t22\tFC\tFF\tFF\tFF\t66\r\n      4644  0CF103A7   00000004    8        17\t1F\t08\t60\tB1\t1F\t08\t66\r\n      4644  0C3C4D4A   00000004    8        BE\tFF\tFF\t7F\t18\tFF\tFF\t66\r\n      4643  0CF102A7   00000004    8        30\t75\tE0\t2E\t80\tFF\tFF\tFD\r\n      4642  0CF101A7   00000004    8        68\t00\t97\tCC\t00\t19\t39\t02\r\n      4642  18F11FF0   00000004    8        FF\t3F\t90\t68\t88\t1B\t10\t6C\r\n      4632  1FFFFFFF   00000004    8        00\t00\tFF\tFF\tFF\tFF\tFF\tFF\r\n      4623  0CF102A7   00000004    8        30\t75\tE0\t2E\t80\tFF\tFF\tFD\r\n      4623  0CF101A7   00000004    8        68\t00\t97\tCC\t00\t19\t39\t01\r\n      4622  1FFFFFFF   00000004    8        00\t00\tFF\tFF\tFF\tFF\tFF\tFF\r\n      4646  18F106A7   00000004    8        00\tF7\tFF\tFF\tFF\tFF\tFF\tCD\r\n      4645  0CF105A7   00000004    8        94\t11\t00\t55\tFF\tFF\tFF\t23\r\n      4645  0CF104A7   00000004    8        F0\t60\t22\tFC\tFF\tFF\tFF\t66\r\n      4644  0CF103A7   00000004    8        17\t1F\t08\t60\tB1\t1F\t08\t66\r\n      4644  0C3C4D4A   00000004    8        BE\tFF\tFF\t7F\t18\tFF\tFF\t66\r\n      4643  0CF102A7   00000004    8        30\t75\tE0\t2E\t80\tFF\tFF\tFD\r\n      4642  0CF101A7   00000004    8        68\t00\t97\tCC\t00\t19\t39\t02\r\n      4642  18F11FF0   00000004    8        FF\t3F\t90\t68\t88\t1B\t10\t6C\r\n      4632  1FFFFFFF   00000004    8        00\t00\tFF\tFF\tFF\tFF\tFF\tFF\r\n      4623  0CF102A7   00000004    8        30\t75\tE0\t2E\t80\tFF\tFF\tFD\r\n      4623  0CF101A7   00000004    8        68\t00\t97\tCC\t00\t19\t39\t01\r\n      4646  18F108A7   00000004    8        F0\t00\t00\tFF\tFF\tFF\tFF\t47\r\n      4646  18F106A7   00000004    8        00\tF7\tFF\tFF\tFF\tFF\tFF\tCD\r\n      4645  0CF105A7   00000004    8        94\t11\t00\t55\tFF\tFF\tFF\t23\r\n      4645  0CF104A7   00000004    8        F0\t60\t22\tFC\tFF\tFF\tFF\t66\r\n      4644  0CF103A7   00000004    8        17\t1F\t08\t60\tB1\t1F\t08\t66\r\n      4644  0C3C4D4A   00000004    8        BE\tFF\tFF\t7F\t18\tFF\tFF\t66\r\n      4643  0CF102A7   00000004    8        30\t75\tE0\t2E\t80\tFF\tFF\tFD\r\n      4642  0CF101A7   00000004    8        68\t00\t97\tCC\t00\t19\t39\t02\r\n      4642  18F11FF0   00000004    8        FF\t3F\t90\t68\t88\t1B\t10\t6C\r\n      4632  1FFFFFFF   00000004    8        00\t00\tFF\tFF\tFF\tFF\tFF\tFF\r\n      4623  0CF102A7   00000004    8        30\t75\tE0\t2E\t80\tFF\tFF\tFD\r\n      4647  18F120F0   00000004    8        2B\t75\t60\tB1\tB0\t01\tFF\tFF\r\n      4646  18F108A7   00000004    8        F0\t00\t00\tFF\tFF\tFF\tFF\t47\r\n      4646  18F106A7   00000004    8        00\tF7\tFF\tFF\tFF\tFF\tFF\tCD\r\n      4645  0CF105A7   00000004    8        94\t11\t00\t55\tFF\tFF\tFF\t23\r\n      4645  0CF104A7   00000004    8        F0\t60\t22\tFC\tFF\tFF\tFF\t66\r\n      4644  0CF103A7   00000004    8        17\t1F\t08\t60\tB1\t1F\t08\t66\r\n      4644  0C3C4D4A   00000004    8        BE\tFF\tFF\t7F\t18\tFF\tFF\t66\r\n      4643  0CF102A7   00000004    8        30\t75\tE0\t2E\t80\tFF\tFF\tFD\r\n      4642  0CF101A7   00000004    8        68\t00\t97\tCC\t00\t19\t39\t02\r\n      4642  18F11FF0   00000004    8        FF\t3F\t90\t68\t88\t1B\t10\t6C\r\n      4632  1FFFFFFF   00000004    8        00\t00\tFF\tFF\tFF\tFF\tFF\tFF\r\n      4648  18F121F0   00000004    8        09\t34\t00\t00\tFF\tFF\tB0\t01\r\n      4647  18F120F0   00000004    8        2B\t75\t60\tB1\tB0\t01\tFF\tFF\r\n      4646  18F108A7   00000004    8        F0\t00\t00\tFF\tFF\tFF\tFF\t47\r\n      4646  18F106A7   00000004    8        00\tF7\tFF\tFF\tFF\tFF\tFF\tCD\r\n      4645  0CF105A7   00000004    8        94\t11\t00\t55\tFF\tFF\tFF\t23\r\n      4645  0CF104A7   00000004    8        F0\t60\t22\tFC\tFF\tFF\tFF\t66\r\n      4644  0CF103A7   00000004    8        17\t1F\t08\t60\tB1\t1F\t08\t66\r\n      4644  0C3C4D4A   00000004    8        BE\tFF\tFF\t7F\t18\tFF\tFF\t66\r\n      4643  0CF102A7   00000004    8        30\t75\tE0\t2E\t80\tFF\tFF\tFD\r\n      4642  0CF101A7   00000004    8        68\t00\t97\tCC\t00\t19\t39\t02\r\n      4642  18F11FF0   00000004    8        FF\t3F\t90\t68\t88\t1B\t10\t6C\r\n      4648  18FB01A7   00000004    8        FF\t1F\tFF\tFF\tFF\tFF\tFF\tFF\r\n      4648  18F121F0   00000004    8        09\t34\t00\t00\tFF\tFF\tB0\t01\r\n      4647  18F120F0   00000004    8        2B\t75\t60\tB1\tB0\t01\tFF\tFF\r\n      4646  18F108A7   00000004    8        F0\t00\t00\tFF\tFF\tFF\tFF\t47\r\n      4646  18F106A7   00000004    8        00\tF7\tFF\tFF\tFF\tFF\tFF\tCD\r\n      4645  0CF105A7   00000004    8        94\t11\t00\t55\tFF\tFF\tFF\t23\r\n      4645  0CF104A7   00000004    8        F0\t60\t22\tFC\tFF\tFF\tFF\t66\r\n      4644
